vi "Tick Count with Error Wires.vi"(10 "error in (no error)":errorcluster) -> (2 "error out":errorcluster, 5 "millisecond timer value":u32)   [LabVIEW 2013, in "WebSockets.lvlib" / "WebSocket.lvclass"]
uses:
  WebSocket/WebSocket.lvclass
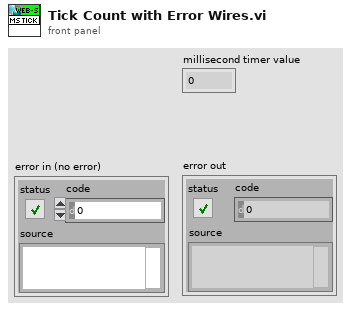
[diagram p1: front panel]
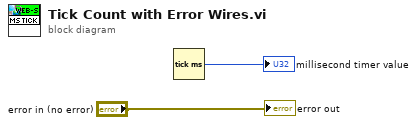
[diagram p0: block diagram]
diagram:
  n1 = Tick Count (ms)() -> (millisecond timer value=→"millisecond timer value":u32)
  "error out" <- "error in (no error)"
